vi "GenerateIOSamplePulseMerge.vi"   [LabVIEW 2017]
doc: "Initiates a pulse on the sample clock terminal of the I/O items."
uses:
  <vilib>/eio/EIOGrowableMethodNode/genericMethod/EIOGrowableMethodNode.xnode
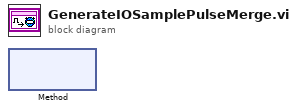
[diagram p0: block diagram]
diagram:
  n1 = xnode " Method"() -> ()  [unwired: 1 in, 1 out]
